vi "Day 5.vi"() -> ()   [LabVIEW 2019]
panel:
  out "Redux Polymer":string
  out "Error Out":errorcluster
  out "Length of Shortest Polymer":i32
  out "Element Creating Shortest Polymer":string
  out "Polymer Length":i32
  out "Polymer After Reacting":string
  in  "error in (no error)":errorcluster
  in  "Use Example Input":bool
  in  "Example Input":string="dabAcCaCBAcCcaDA"
  in  "Relative Path to Input File":string="Day 5\\Day 5 Raw Input.txt"
  # "Part 1"
  # "Part 2"
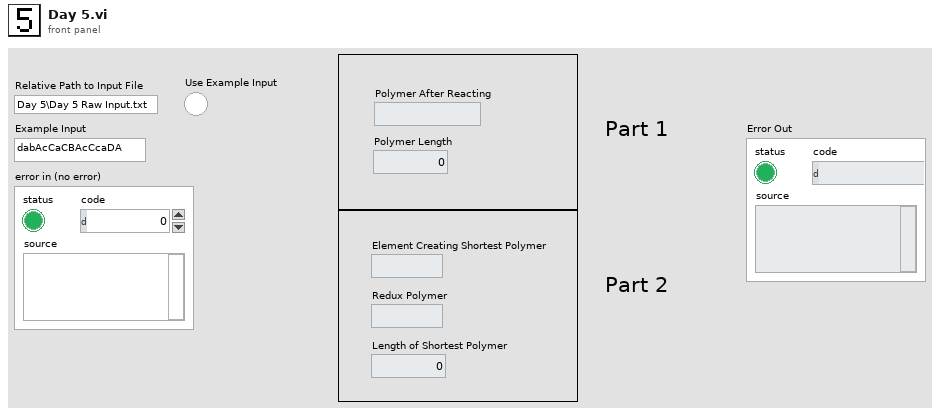
[diagram p1: front panel]
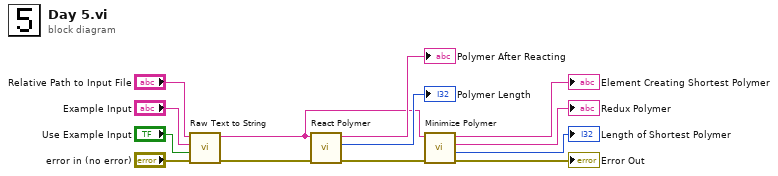
[diagram p0: block diagram]
diagram:
  n1 = call "Raw Text to String.vi"("Error In"="error in (no error)", "Use Example Input"="Use Example Input", "Example Input"="Example Input", "Relative Path to Input File"="Relative Path to Input File") -> ("Error Out"=w7:errorcluster, "String"=w6:string)  [unwired: 6 in]
  n2 = call "React Polymer.vi"("Error In"=w7, "Unreacted Polymer"=w6) -> ("Error Out"=w4:errorcluster, "Size of Polymer"=→"Polymer Length":i32, "Polymer"=→"Polymer After Reacting":string)  [unwired: 7 in]
  n3 = call "Minimize Polymer.vi"("Error In"=w4, "Unreacted Polymer"=w6) -> ("Error Out"=→"Error Out":errorcluster, "Size of Redux Polymer"=→"Length of Shortest Polymer":i32, "Redux Polymer"=→"Redux Polymer":string, "Redux Element"=→"Element Creating Shortest Polymer":string)  [unwired: 6 in]
